vi "Hyperbolic Cosine Integral.vi"(3 "x":dbl format="%.2f") -> (1 "Chi(x)":dbl format="%.2f")   [LabVIEW 2017, in "NI_Gmath.lvlib"]
doc: "Computes the hyperbolic cosine integral function."
uses:
  <vilib>/gmath/NI_Gmath.lvlib
  <resource>/lvanlys.dll
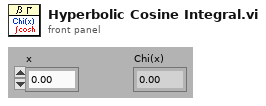
[diagram p1: front panel]
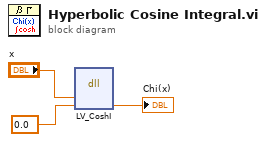
[diagram p0: block diagram]
diagram:
  n1 = dll-call lib="e:/builds/penguin/labview/branches/2017/dev/dist/resource/lvanlys.*" fn="LV_CoshI"("x"="x", "CoshI(x)"=0.0 ("cosI")) -> ("CoshI(x)"=→"Chi(x)":dbl)  [unwired: 5 in, 2 out]
